vi "Get Channel Data.vi"(8 "error in":errorcluster, 11 "Channel in":refnum<class "Channel.lvclass">) -> (0 "error out":errorcluster, 2 "Channel Data":T1, 3 "Channel out":refnum<class "Channel.lvclass">)   [LabVIEW 2024, in "Parser.lvlib" / "Channel.lvclass"]
uses:
  Channel.lvclass
  Channel.lvclass/Channel.ctl
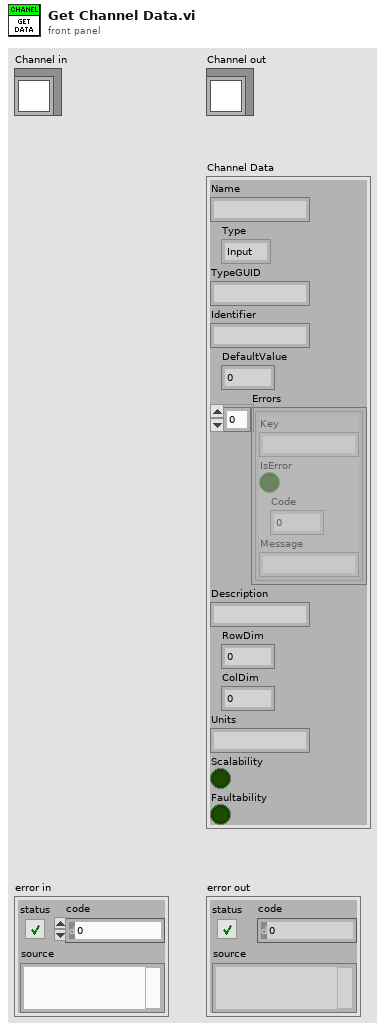
[diagram p1: front panel]
types:
  T1 = cluster{"Name":string, "Type":enum16{"Input", "Output"}, "TypeGUID":string, "Identifier":string, "DefaultValue":dbl, "Errors":cluster{"Key":string, "IsError":bool, "Code":u32, "Message":string}[], "Description":string, "RowDim":i32, "ColDim":i32, "Units":string, "Scalability":bool, "Faultability":bool}
  T2 = cluster{"Key":string, "IsError":bool, "Code":u32, "Message":string}[]
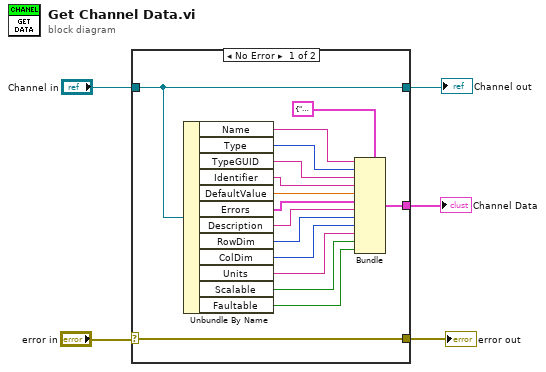
[diagram p0: block diagram]
diagram:
  n1 = case shown="No Error" "error in" {
    selector: "error in" -> [w21 w23]
    tunnel: [w20 _] -> w3
    tunnel: "Channel in" -> [w6 w22]
    tunnel: [w21 w23] -> w4
    tunnel: [w6 w22] -> w1
    frame No Error {
      n2 = Unbundle By Name(w6) -> ("Name"=w19:string, "Type"=w18:enum16{"Input", "Output"}, "TypeGUID"=w17:string, "Identifier"=w16:string, "DefaultValue"=w15:dbl, "Errors"=w14:T2, "Description"=w13:string, "RowDim"=w12:i32, "ColDim"=w11:i32, "Units"=w10:string, "Scalable"=w9:bool, "Faultable"=w8:bool)
      n3 = Bundle(cluster=T1 {"Name"="", "Type"=enum."Input", "TypeGUID"="", "Identifier"="", "DefaultValue"=0.0, "Errors"=[], "Description"="", "RowDim"=0, "ColDim"=0, "Units"="", "Scalability"=FALSE, "Faultability"=FALSE}, "Name"=w19, "Type"=w18, "TypeGUID"=w17, "Identifier"=w16, "DefaultValue"=w15, "Errors"=w14, "Description"=w13, "RowDim"=w12, "ColDim"=w11, "Units"=w10, "Scalability"=w9, "Faultability"=w8) -> (w20:T1)
    }
    frame Error {
    }
  }
  "error out" <- w4
  "Channel Data" <- w3
  "Channel out" <- w1
